vi "Read Frame File.vi"() -> ()   [LabVIEW 2013]
uses:
  <vilib>/Utility/file.llb/Read From Spreadsheet File (I64).vi
panel:
  out "data 2":dbl[](graph)
  out "Address":i16[](array[numeric])
  out "Array":i32[](array[numeric])
  out "x .and. y?":i32[][](graph)
  out "data":i16[](graph)
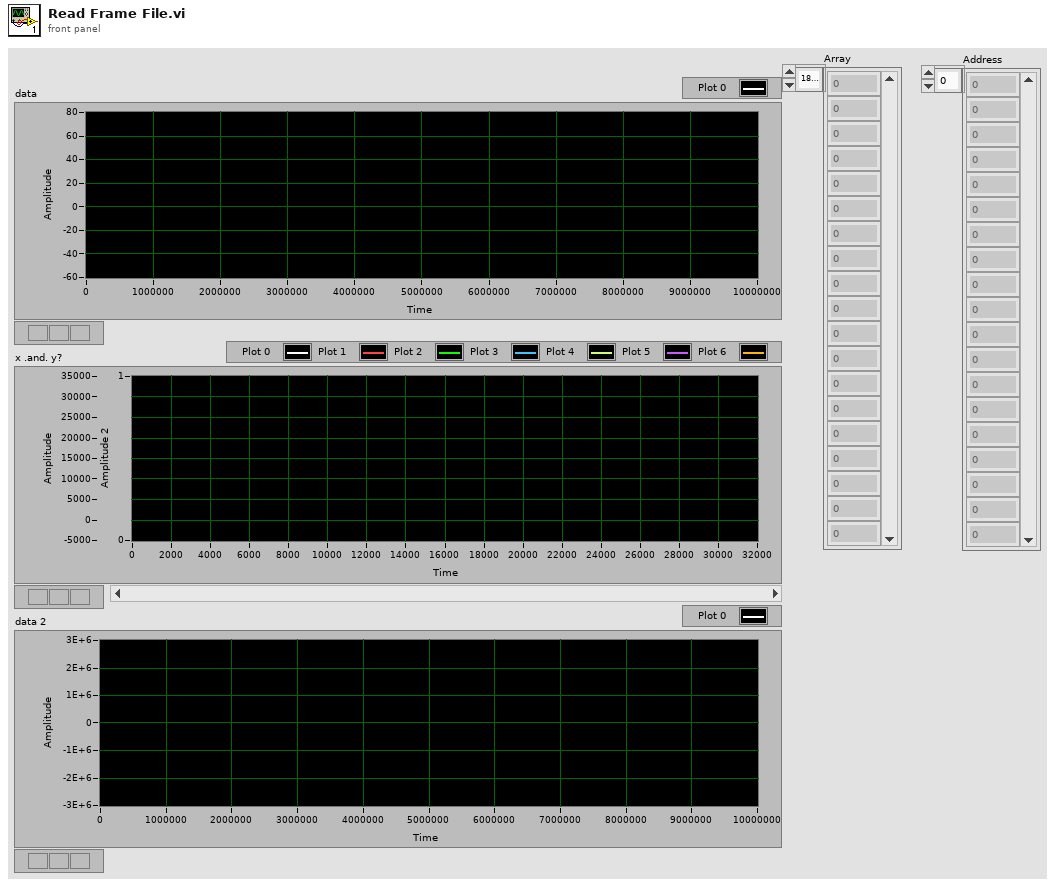
[diagram p1: front panel]
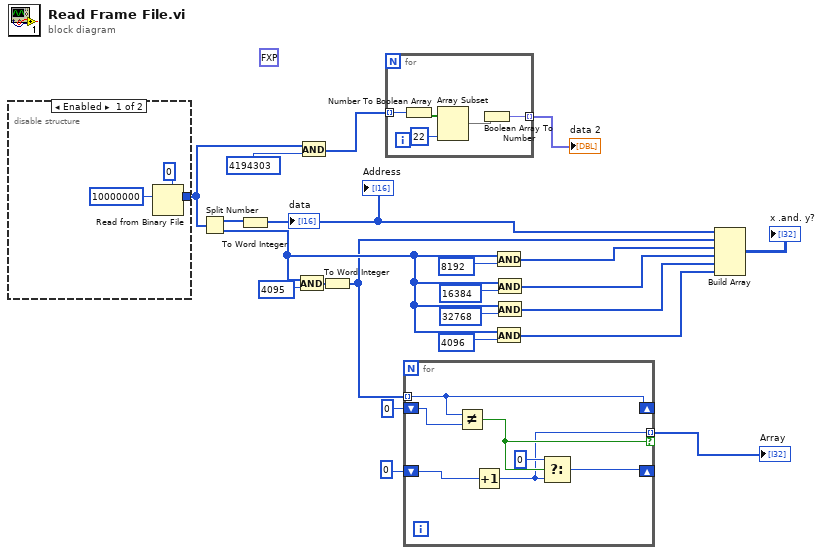
[diagram p0: block diagram]
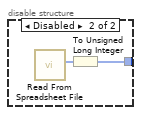
[diagram p2: hidden frame]
diagram:
  (unwired) fxp<+/-,22,22> 0.0 ("Fixed")
  n1 = disable-structure shown="Enabled" {
    disable-tunnel: [w23 w26] -> w3
    frame Enabled {
      n2 = Read from Binary File(5:u32 0, 10:10000000 ("count (1)")) -> (2:w23:u32[])  [unwired: 4 in, 3 out]
    }
    frame Disabled {
      n3 = call-poly <vilib>:"Read From Spreadsheet File.vi"() -> ("first row"=w27:i64[])  [unwired: 7 in, 4 out]
      n4 = To Unsigned Long Integer(number=w27) -> (unsigned 32bit integer=w26:u32[])
    }
  }
  n5 = Split Number(x=w3) -> (hi(x)=w22:u16[], lo(x)=w7:u16[])
  n6 = To Word Integer(number=w22) -> (16bit integer=w16:i16[])
  "data" <- w16
  "Address" <- w16
  n7 = And(x=w7, y=4095) -> (x .and. y?=w18:i32[])
  n8 = And(x=w3, y=u32 4194303) -> (x .and. y?=w2:u32[])
  n9 = To Word Integer(number=w18) -> (16bit integer=w5:i16[])
  n10 = for {
    tunnel: w2 -> [w32] mode=indexing
    tunnel: [w28] -> w1 mode=indexing
    n11 = Number To Boolean Array(number=w32) -> (Boolean array=w31:bool[])
    n12 = Array Subset(array=w31, length=22) -> (w29:bool[])  [unwired: 1 in]
    n13 = Boolean Array To Number(Boolean array=w29) -> (number=w28:fxp<+/-,22,22>)
  }
  "data 2" <- w1
  n14 = for {
    tunnel: w5 -> [w39] mode=indexing
    shift-right: [w39] -> _
    shift-left: 0 -> [w38]
    shift-right: [w34] -> _
    shift-left: 0 -> [w37]
    tunnel: [w33] -> w17 mode=indexing if=w35
    n15 = Not Equal?(x=w39, y=w38) -> (x != y?=w35:bool)
    n16 = Increment(x=w37) -> (x+1=w33:i32)
    n17 = Select(t=0, s=w35, f=w33) -> (s? t:f=w34:i32)
  }
  "Array" <- w17
  n18 = And(x=w7, y=8192) -> (x .and. y?=w12:i32[])
  n19 = And(x=w7, y=4096) -> (x .and. y?=w6:i32[])
  n20 = And(x=w7, y=16384) -> (x .and. y?=w11:i32[])
  n21 = And(x=w7, y=32768) -> (x .and. y?=w9:i32[])
  n22 = Build Array(w16, w5, w12, w11, w9, w6) -> (→"x .and. y?":i32[][])
